vi "setImageDST.vi"(8 "error in (no error)":errorcluster, 10 "Image":T1, 11 "ax5 in":refnum<class "ax5.lvclass">) -> (0 "error out":errorcluster, 3 "ax5 out":refnum<class "ax5.lvclass">)   [LabVIEW 2017, in "ax5.lvclass"]
uses:
  ax5.lvclass
  <vilib>/vision/Image Controls.llb/IMAQ Image.ctl
  ax5.lvclass/ax5.ctl
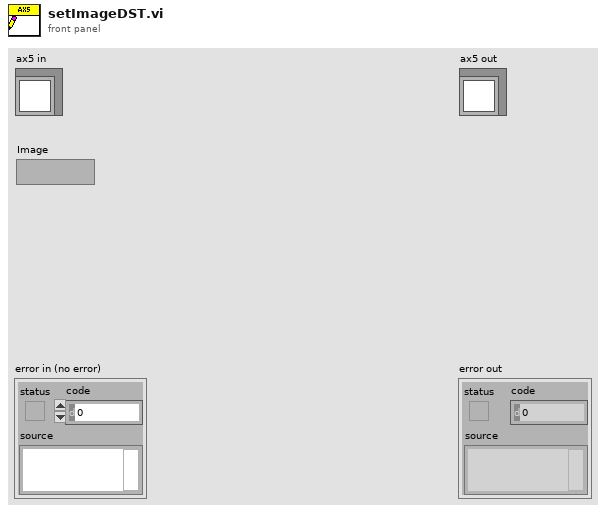
[diagram p1: front panel]
types:
  T1 = typedef "IMAQ Image.ctl" = refnum<image>
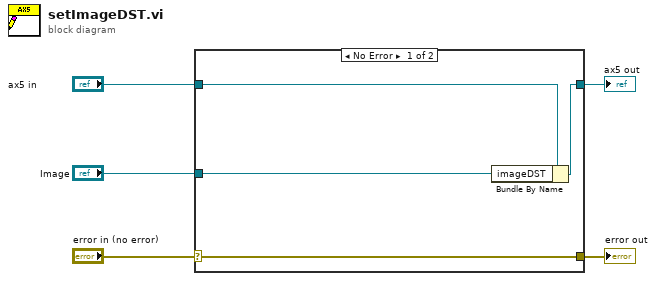
[diagram p0: block diagram]
diagram:
  n1 = case shown="No Error" "error in (no error)" {
    selector: "error in (no error)" -> [w9 w10]
    tunnel: [w9 w10] -> w4
    tunnel: [w7 w11] -> w2
    tunnel: "ax5 in" -> [w8 w11]
    tunnel: "Image" -> [w6 _]
    frame No Error {
      n2 = Bundle By Name(cluster=w8, "imageDST"=w6) -> (w7:refnum<class "ax5.lvclass">)
    }
    frame Error {
    }
  }
  "error out" <- w4
  "ax5 out" <- w2
